vi "WSVCAP SHL Host LL RFFE Build and Parse Data.vi"(0 "Data Out":string, 1 "Data Out (Cycle Commands)":string[](array[string]), 2 "Post Command Delay":dbl[](array[numeric]) format="%#.0p s", 5 "Data Out (Unique)":string[](array[string]), 7 "Clock Rate (Hz) (Cycle Only)":dbl=50000.0, 9 "RFFE Data In [U8]":u8[][](array[numeric]) format="%02x", 12 "Simulate FPGA (Cycle Only)":bool, 13 "DUT Mask (All)":bool[](array[boolean])=[TRUE, TRUE, TRUE, TRUE, TRUE, TRUE, TRUE, TRUE, TRUE, TRUE, TRUE, TRUE, TRUE, TRUE, TRUE, TRUE]) -> (4 "RFFE Data Out [U8]":u8[][](array[numeric]) format="%02x", 6 "CMD Lengths (Bits)":u8[](array[numeric]), 8 "CMD Delays (Ticks)":u32[](array[numeric]), 10 "RFFE Data In":string[](array[string]))   [LabVIEW 2012]
panel:
  # "DUT 01"
  # "DUT 02"
  # "DUT 03"
  # "DUT 04"
  # "DUT 05"
  # "DUT 06"
  # "DUT 07"
  # "DUT 08"
  # "DUT 09"
  # "DUT 10"
  # "DUT 11"
  # "DUT 12"
  # "DUT 13"
  # "DUT 14"
  # "DUT 15"
  # "DUT 16"
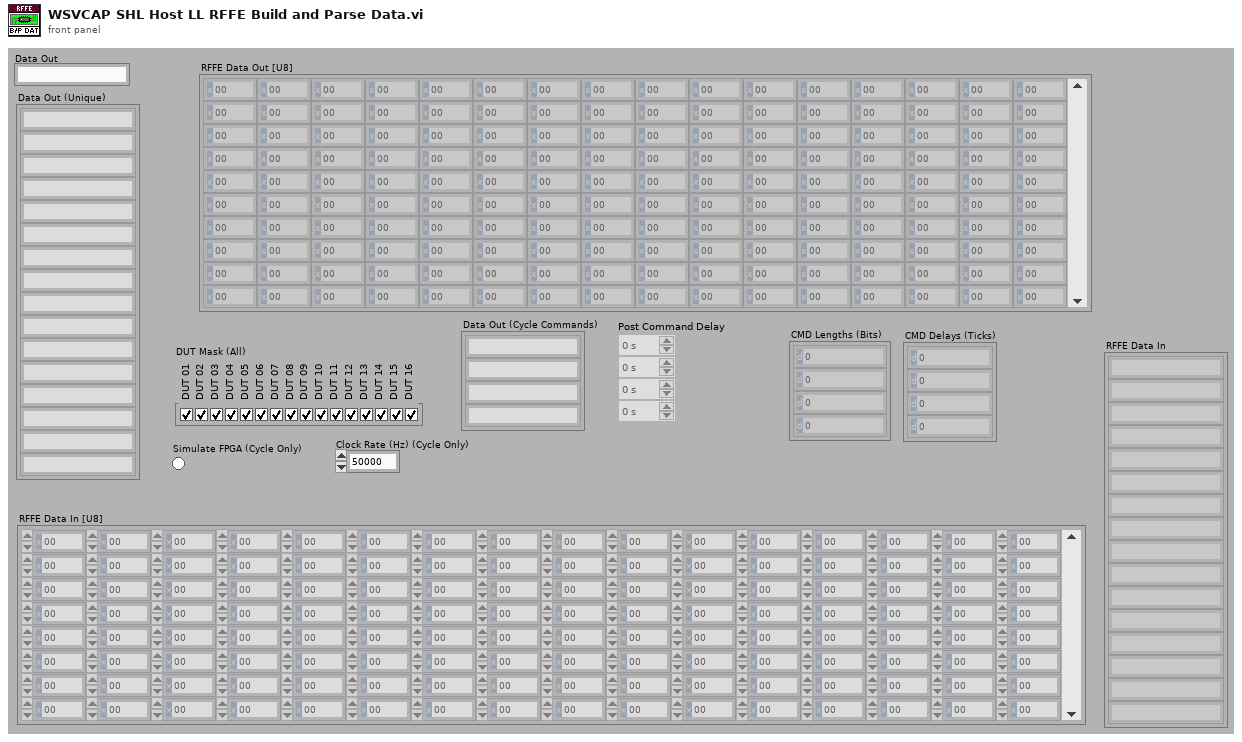
[diagram p1: front panel]
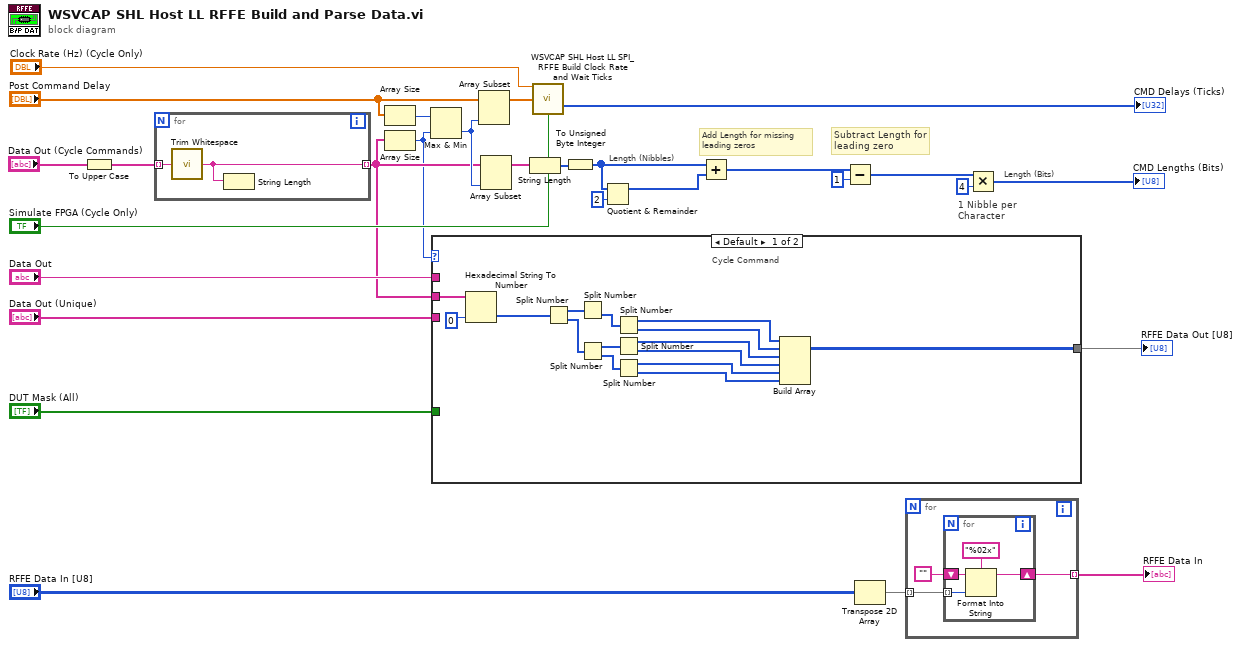
[diagram p0: block diagram]
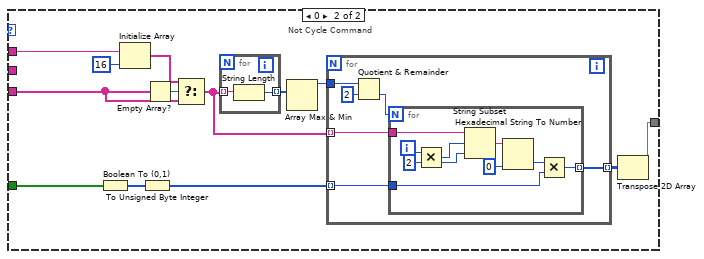
[diagram p2: hidden frame]
diagram:
  # "Subtract Length for\nleading zero"
  # "Add Length for missing\nleading zeros"
  # "Length (Bits)"
  # "Length (Nibbles)"
  # "1 Nibble per Character"
  n1 = To Upper Case(1:"Data Out (Cycle Commands)") -> (0:w1:string[])
  n2 = for {
    tunnel: w1 -> [w30] mode=indexing
    tunnel: [w29] -> w12 mode=indexing
    n3 = call <vilib>:"Trim Whitespace.vi"("string"=w30) -> ("trimmed string"=w29:string)  [unwired: 1 in]
    n4 = String Length(string=w29) -> ()  [unwired: 1 out]
  }
  n5 = Array Size(array="Post Command Delay") -> (size(s)=w21:i32)
  n6 = Array Size(array=w12) -> (size(s)=w11:i32)
  n7 = Max & Min(x=w21, y=w11) -> (min(x,y)=w18:i32)  [unwired: 1 out]
  n8 = case shown="Default" w11 {
    tunnel: "DUT Mask (All)" -> [_ w58]
    tunnel: "Data Out (Unique)" -> [_ w51]
    tunnel: [w37 w50] -> w24
    tunnel: "Data Out" -> [_ w46]
    tunnel: w12 -> [w45 _]
    frame Default {
      # "Cycle Command"
      n9 = Hexadecimal String To Number(string=w45, default (0uL)=u64 0 ("Read Data")) -> (number=w38:u64[])  [unwired: 1 in, 1 out]
      n10 = Split Number(x=w38) -> (hi(x)=w43:u32[], lo(x)=w42:u32[])
      n11 = Split Number(x=w43) -> (lo(x)=w41:u16[])  [unwired: 1 out]
      n12 = Split Number(x=w42) -> (hi(x)=w40:u16[], lo(x)=w39:u16[])
      n13 = Split Number(x=w41) -> (hi(x)=w31:u8[], lo(x)=w36:u8[])
      n14 = Split Number(x=w40) -> (hi(x)=w35:u8[], lo(x)=w34:u8[])
      n15 = Split Number(x=w39) -> (hi(x)=w33:u8[], lo(x)=w32:u8[])
      n16 = Build Array(w31, w36, w35, w34, w33, w32) -> (w37:u8[][])
    }
    frame 0 {
      # "Not Cycle Command"
      n17 = Boolean To (0,1)(Boolean=w58) -> (0, 1=w57:i16[])
      n18 = Initialize Array(w46, 16 ("dimension size")) -> (w52:string[])
      n19 = To Unsigned Byte Integer(number=w57) -> (unsigned 8bit integer=w56:u8[])
      n20 = Empty Array?(array=w51) -> (empty?=w54:bool)
      n21 = Select(t=w52, s=w54, f=w51) -> (s? t:f=w49:string[])
      n22 = for {
        tunnel: w49 -> [w60] mode=indexing
        tunnel: [w59] -> w48 mode=indexing
        n23 = String Length(string=w60) -> (length=w59:i32)
      }
      n24 = Array Max & Min(array=w48) -> (max value=w47:i32)  [unwired: 3 out]
      n25 = for {
        tunnel: w56 -> [w64] mode=indexing
        tunnel: [w63] -> w55 mode=indexing
        tunnel: w49 -> [w62] mode=indexing
        tunnel: w47 -> [w61]
        n26 = Quotient & Remainder(x=w61, y=2) -> (floor(x/y)=w65:i32)  [unwired: 1 out]
        n27 = for {
          N: w65 -> [_]
          tunnel: w62 -> [w75]
          tunnel: [w68] -> w63 mode=indexing
          tunnel: w64 -> [w69]
          i -> [w74]
          w72 = 2 ("y")
          n28 = Multiply(x=w74, y=w72) -> (x*y=w73:i32)
          n29 = String Subset(string=w75, offset (0)=w73, length (rest)=w72) -> (substring=w71:string)
          n30 = Hexadecimal String To Number(string=w71, default (0uL)=u8 0 ("default (0 U32)")) -> (number=w67:u8)  [unwired: 1 in, 1 out]
          n31 = Multiply(x=w67, y=w69) -> (x*y=w68:u8)
        }
      }
      n32 = Transpose 2D Array(2D array=w55) -> (transposed array=w50:u8[][])
    }
  }
  "RFFE Data Out [U8]" <- w24
  n33 = Array Subset(array="Post Command Delay", length=w18) -> (w19:dbl[])  [unwired: 1 in]
  n34 = Array Subset(array=w12, length=w18) -> (w17:string[])  [unwired: 1 in]
  n35 = String Length(string=w17) -> (length=w23:i32[])
  n36 = call "WSVCAP SHL Host LL SPI_RFFE Build Clock Rate and Wait Ticks.vi"("Clock Rate (Hz)"="Clock Rate (Hz) (Cycle Only)", "CMD Delay (s)"=w19, "Simulate FPGA"="Simulate FPGA (Cycle Only)") -> ("CMD Delay (Ticks)"=→"CMD Delays (Ticks)":u32[])  [unwired: 9 in, 3 out]
  n37 = To Unsigned Byte Integer(number=w23) -> (unsigned 8bit integer=w8:u8[])
  n38 = Quotient & Remainder(x=w8, y=u8 2) -> (x-y*floor(x/y)=w7:u8[])  [unwired: 1 out]
  n39 = Add(x=w8, y=w7) -> (x+y=w5:u8[])
  n40 = Subtract(x=w5, y=u8 1 ("Read Data")) -> (x-y=w3:u8[])
  n41 = Transpose 2D Array(2D array="RFFE Data In [U8]") -> (transposed array=w27:u8[][])
  n42 = for {
    tunnel: w27 -> [w78] mode=indexing
    tunnel: [w76] -> w26 mode=indexing
    n43 = for {
      tunnel: w78 -> [w82] mode=indexing
      shift-right: [w80] -> w76
      shift-left: "" -> [w79]
      n44 = Format Into String(format string="%02x", initial string=w79, w82) -> (resulting string=w80:string)  [unwired: 1 in, 1 out]
    }
  }
  "RFFE Data In" <- w26
  n45 = Multiply(x=w3, y=u8 4 ("Read Data")) -> (x*y=→"CMD Lengths (Bits)":u8[])
